vi "Open Property.vi"   [LabVIEW 2015, in "SLSC Interface.lvclass"]
uses:
  SLSC Interface.lvclass
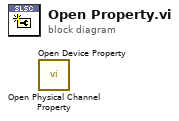
[diagram p0: block diagram]
diagram:
  n1 = call "Open Physical Channel Property.vi"() -> ()  [unwired: 13 in, 3 out]
  n2 = call "Open Device Property.vi"() -> ()  [unwired: 13 in, 3 out]
